vi "Interface - Inheritance.vi"(7 "Msg Chain":string, 8 "error in (no error)":errorcluster {"code" format="Error %.0f"}, 10 "Interfaces":refnum<class "Interface Documenation.lvclass">[](array[class]), 11 "VIDoc Printer - Confluence In":refnum<class "VIDoc Printer - Confluence.lvclass">) -> (0 "error out":errorcluster {"code" format="Error %.0f"}, 3 "VIDoc Printer - Confluence Out":refnum<class "VIDoc Printer - Confluence.lvclass">)   [LabVIEW 2023, in "VIDoc Printer - Confluence.lvlib" / "VIDoc Printer - Confluence.lvclass"]
uses:
  VIDoc Printer - Confluence.lvclass
  C:/projects/DMC/Tooling/Git-Action-Service/Source/Documentation Generation/Printers/Printer/VIDoc Printer.lvclass
  Parsing/Interface Documenation/Interface Documenation.lvclass
  Parsing/Interface Documenation/Interface Documenation.lvclass/Interface Documenation.ctl
  Confluence Formatting/Types/Format Combo Box.ctl
  Parsing/Interface Documenation/Get Parent Interfaces.vi
  Parsing/Interface Documenation/Get Name.vi
  VIDoc Printer - Confluence.lvclass/VIDoc Printer - Confluence.ctl
  Printer/VIDoc Printer.lvclass
  UI Interaction/UI Interaction.lvclass
  Confluence Formatting/Confluence Formatting.lvlib
  C:/projects/DMC/Tooling/Git-Action-Service/Source/Documentation Generation/Printers/Confluence Printer/VIDoc Printer - Confluence.lvclass
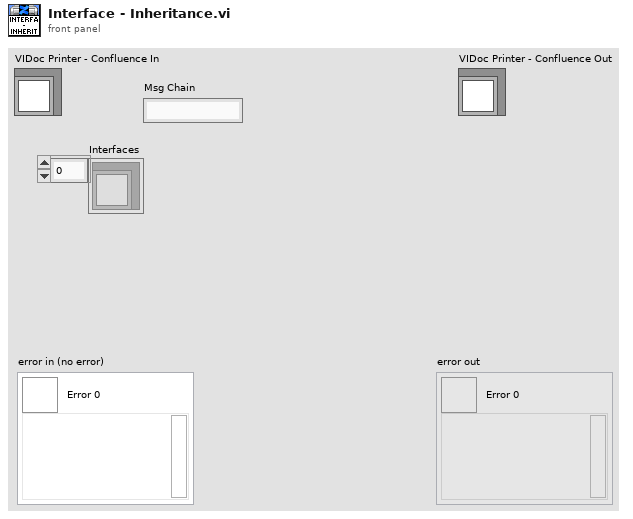
[diagram p1: front panel]
types:
  T1 = typedef "Confluence Formatting.lvlib/Format Combo Box.ctl" = string
  T2 = typedef "VIDoc Parsing.lvlib/Base Class Info Cluster.ctl" = cluster{"Name":string, "Icon":T3, "Version":cluster{"Major":u16, "Minor":u16, "Fix":u16, "Build":u16}, "Description":string, "Friends":string[], "ChildRefsRestricted":bool, "TransferMustOverrides":bool, "Path":path, "Qualified Name":string, "Class Scope":enum32{"invalid scope", "public", "private", "protected", "community"}}
  T3 = typedef "imagedata.ctl" = cluster{"image type":i32, "image depth":i32, "image":u8[], "mask":u8[], "colors":u32[], "Rectangle":cluster{"left":i16, "top":i16, "right":i16, "bottom":i16}}
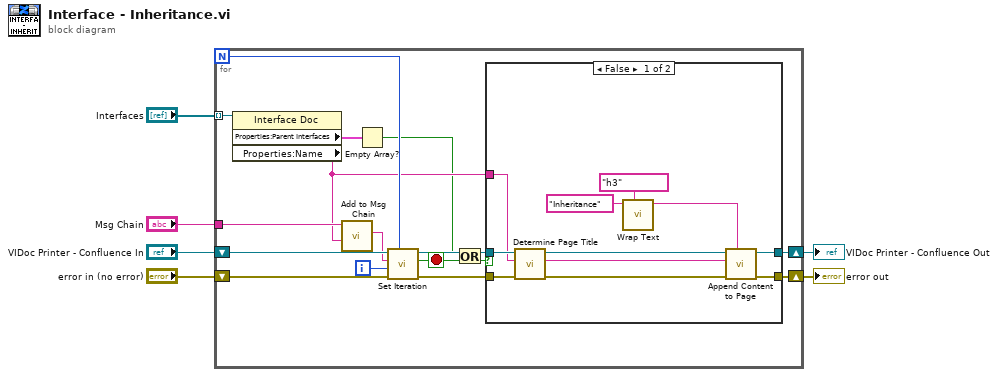
[diagram p0: block diagram]
diagram:
  n1 = for {
    N -> [w15]
    shift-right: [w20] -> w6
    shift-left: "error in (no error)" -> [w18]
    shift-right: [w21] -> w5
    shift-left: "VIDoc Printer - Confluence In" -> [w19]
    tunnel: "Interfaces" -> [w22] mode=indexing
    tunnel: "Msg Chain" -> [w13]
    i -> [w14]
    stop <- w10 stop-if-true
    n2 = property class="Interface Doc"(reference=w22) -> ("Properties:Parent Interfaces"=w9:T2[], "Properties:Name"=w12:string)  [unwired: 1 in, 2 out]
    n3 = call "Add to Msg Chain.vi"("New"=w12, "Msg Chain in"=w13) -> ("Msg Chain out"=w11:string)  [unwired: 9 in]
    n4 = Empty Array?(array=w9) -> (empty?=w7:bool)
    n5 = call "Set Iteration.vi"("Progress Max"=w15, "error in (no error)"=w18, "Progress Value"=w14, "Message (No Message Update)"=w11, "VIDoc Printer In"=w19) -> ("error out"=w16:errorcluster, "Abort?"=w10:bool, "VIDoc Printer Out"=w17:refnum<class "VIDoc Printer - Confluence.lvclass">)  [unwired: 4 in]
    n6 = Or(x=w7, y=w10) -> (x .or. y?=w8:bool)
    n7 = case shown="False" w8 {
      tunnel: [w30 w34] -> w21
      tunnel: [w29 w35] -> w20
      tunnel: w17 -> [w27 w34]
      tunnel: w16 -> [w26 w35]
      tunnel: w12 -> [w25 _]
      frame False {
        n8 = call "Determine Page Title.vi"("error in (no error)"=w26, "Name"=w25, "VIDoc Printer - Confluence In"=w27) -> ("error out"=w32:errorcluster, "Page Title"=w33:string, "VIDoc Printer - Confluence Out"=w31:refnum<class "VIDoc Printer - Confluence.lvclass">)  [unwired: 5 in, 1 out]
        n9 = call "Wrap Text.vi"("Formatting"=T1 "h3", "String"="Inheritance") -> ("Wrapped String"=w23:string)  [unwired: 8 in, 1 out]
        n10 = call "Append Content to Page.vi"("Page Content"=w23, "error in (no error)"=w32, "Page Title"=w33, "VIDoc Printer - Confluence In"=w31) -> ("error out"=w29:errorcluster, "VIDoc Printer - Confluence Out"=w30:refnum<class "VIDoc Printer - Confluence.lvclass">)  [unwired: 6 in]
      }
      frame True {
      }
    }
  }
  "error out" <- w6
  "VIDoc Printer - Confluence Out" <- w5
